vi "Receive Value Change Event.vi"(8 "error in (no error)":errorcluster, 10 "ValueChangeMsg":refnum<class "ValueChangeMsg.lvclass">, 11 "ExampleViewManager In":refnum<class "ExampleViewManager.lvclass">) -> (0 "error out":errorcluster, 3 "ExampleViewManager Out":refnum<class "ExampleViewManager.lvclass">)   [LabVIEW 2017, in "MVA Example.lvlib" / "ExampleViewManager.lvclass"]
doc: "<License>\nCopyright © 2017 Composed Systems, LLC | All rights reserved\nwww.composed.io\n\nAuthor: Ethan Stern <ethan.stern@composed.io>\n\nThis software is provided \"AS IS\" WITHOUT WARRANTIES, either express or implied, AND IS FOR EDUCATIONAL PURPOSES ONLY.\n</License>MVA Framework 1.6.0.31\nEthan Stern - Composed Systems\nCopyright (c) 2018, Composed Systems"
uses:
  ExampleViewManager.lvclass
  <vilib>/Composed Systems/MVA Framework/Framework/ActorEvents/IEventAggregator Messages/ValueChangeMsg/ValueChangeMsg.lvclass
  <vilib>/Composed Systems/MVA Framework/Framework/ActorEvents/IEventAggregator Messages/ValueChangeMsg/ValueChangeMsg.lvclass/ValueChangeMsg.ctl
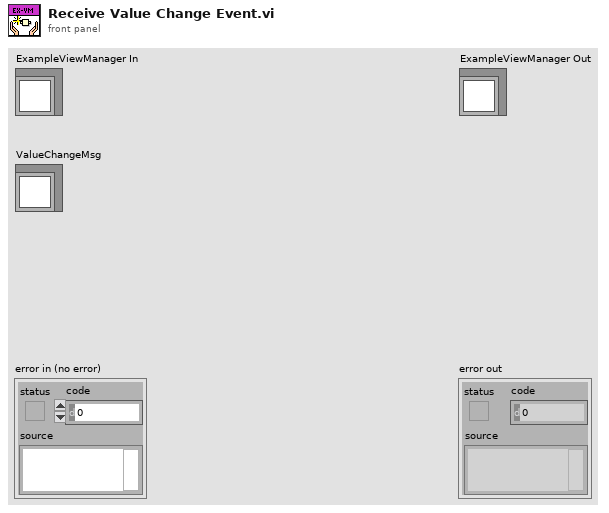
[diagram p1: front panel]
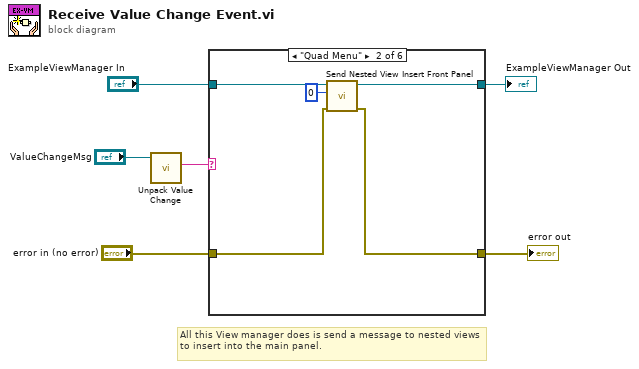
[diagram p0: block diagram]
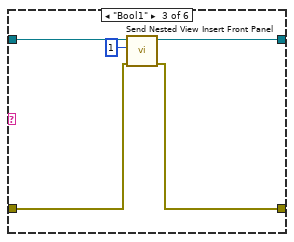
[diagram p3: hidden frame]
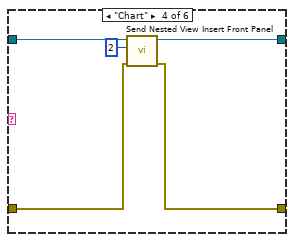
[diagram p4: hidden frame]
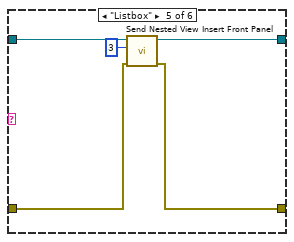
[diagram p5: hidden frame]
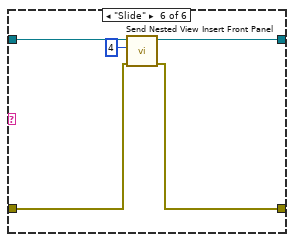
[diagram p6: hidden frame]
diagram:
  # "All this View manager does is send a message to nested views to insert into the main panel."
  n1 = call <vilib>:"Unpack Value Change.vi"("ValueChangeMsg"="ValueChangeMsg") -> ("Control Label"=w2:string)  [unwired: 6 in, 4 out]
  n2 = case shown="\"Quad Menu\"" w2 {
    tunnel: "ExampleViewManager In" -> [w8 w13 w18 w23 w28 w33]
    tunnel: [w8 w12 w17 w22 w27 w32] -> w4
    tunnel: "error in (no error)" -> [w7 w11 w16 w21 w26 w31]
    tunnel: [w7 w10 w15 w20 w25 w30] -> w1
    frame "False", Default {
    }
    frame "Quad Menu" {
      n3 = call "Send Nested View Insert Front Panel.vi"("error in (no error)"=w11, "View Index"=0, "ExampleViewManager in"=w13) -> ("error out"=w10:errorcluster, "ExampleViewManager out"=w12:refnum<class "ExampleViewManager.lvclass">)  [unwired: 7 in]
    }
    frame "Bool1" {
      n4 = call "Send Nested View Insert Front Panel.vi"("error in (no error)"=w16, "View Index"=1, "ExampleViewManager in"=w18) -> ("error out"=w15:errorcluster, "ExampleViewManager out"=w17:refnum<class "ExampleViewManager.lvclass">)  [unwired: 7 in]
    }
    frame "Chart" {
      n5 = call "Send Nested View Insert Front Panel.vi"("error in (no error)"=w21, "View Index"=2, "ExampleViewManager in"=w23) -> ("error out"=w20:errorcluster, "ExampleViewManager out"=w22:refnum<class "ExampleViewManager.lvclass">)  [unwired: 7 in]
    }
    frame "Listbox" {
      n6 = call "Send Nested View Insert Front Panel.vi"("error in (no error)"=w26, "View Index"=3, "ExampleViewManager in"=w28) -> ("error out"=w25:errorcluster, "ExampleViewManager out"=w27:refnum<class "ExampleViewManager.lvclass">)  [unwired: 7 in]
    }
    frame "Slide" {
      n7 = call "Send Nested View Insert Front Panel.vi"("error in (no error)"=w31, "View Index"=4, "ExampleViewManager in"=w33) -> ("error out"=w30:errorcluster, "ExampleViewManager out"=w32:refnum<class "ExampleViewManager.lvclass">)  [unwired: 7 in]
    }
  }
  "error out" <- w1
  "ExampleViewManager Out" <- w4
